vi "3_1_conv bet two impulse.vi"() -> ()   [LabVIEW 2009]
uses:
  <vilib>/Analysis/2dsp.llb/1D Convolution (DBL).vi
  <vilib>/Analysis/NI_AALBase.lvlib
  <vilib>/Analysis/NI_AALPro.lvlib
panel:
  in  "Delay of the second impulse":i32
  in  "Delay of the first impulse":i32
  in  "samples":i32=128
  out "conv(x,y)":dbl[](graph)
  out "Sequence y[n]":dbl[](graph)
  out "Sequence x[n]":dbl[](graph)
  # "Program Developed by Indranil Sinharoy"
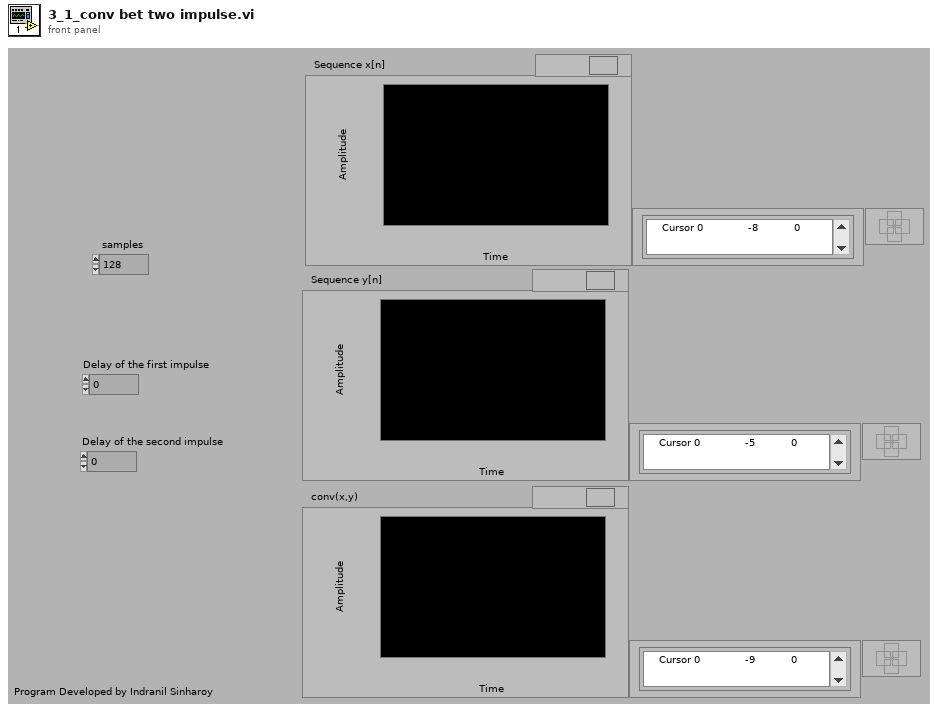
[diagram p1: front panel]
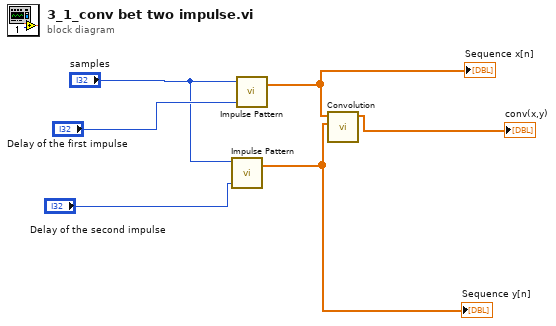
[diagram p0: block diagram]
diagram:
  n1 = call <vilib>:"Impulse Pattern.vi"("delay"="Delay of the second impulse", "samples"="samples") -> ("Impulse Pattern"=w5:dbl[])  [unwired: 1 in, 1 out]
  "Sequence y[n]" <- w5
  n2 = call <vilib>:"Impulse Pattern.vi"("delay"="Delay of the first impulse", "samples"="samples") -> ("Impulse Pattern"=w4:dbl[])  [unwired: 1 in, 1 out]
  "Sequence x[n]" <- w4
  n3 = call-poly <vilib>:"Convolution.vi"("Y"=w5, "X"=w4) -> ("X * Y"=→"conv(x,y)":dbl[])  [unwired: 8 in, 1 out]
